vi "LearnBAGO.vi"(8 "error in (no error)":errorcluster, 11 "AER in":refnum<class "AER.lvclass">) -> (0 "error out":errorcluster, 3 "AER out":refnum<class "AER.lvclass">)   [LabVIEW 2016, in "AER.lvclass"]
uses:
  AER.lvclass
  AER.lvclass/AER.ctl
panel:
  out "size(s)":i32
  in  "gamma":dbl=-3e-05 format="%#_13g"
  out "WBAGO":dbl[](graph)
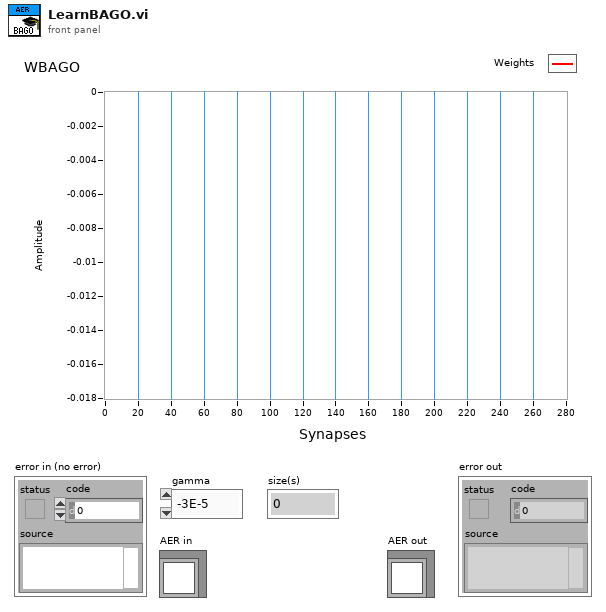
[diagram p1: front panel]
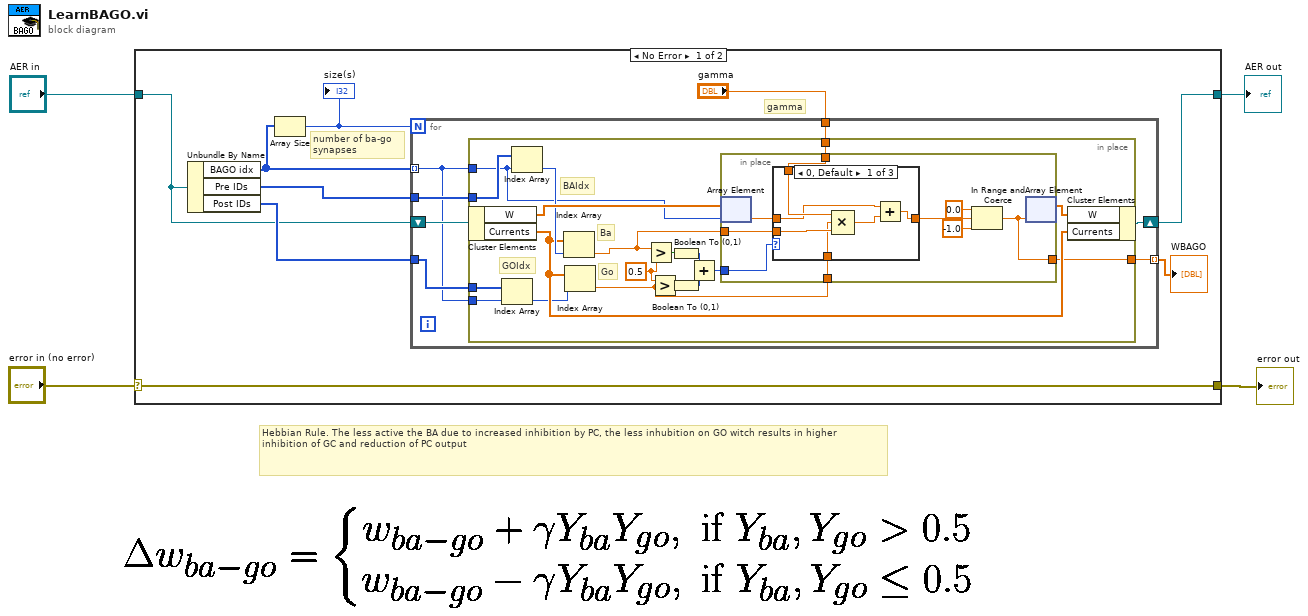
[diagram p0: block diagram]
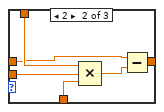
[diagram p2: hidden frame]
diagram:
  # "Hebbian Rule. The less active the BA due to increased inhibition by PC, the less inhubition on GO witch results in higher inhibition of GC and reduction of PC output"
  n1 = case shown="No Error" "error in (no error)" {
    selector: "error in (no error)" -> [w13 w62]
    tunnel: [w13 w62] -> w3
    tunnel: [w7 w63] -> w1
    tunnel: "AER in" -> [w6 w63]
    frame No Error {
      # "gamma"
      # "number of ba-go synapses"
      n2 = Unbundle By Name(w6) -> ("BAGO idx"=w11:i32[], "Pre IDs"=w10:i32[], "Post IDs"=w9:i32[])
      n3 = Array Size(array=w11) -> (size(s)=w12:i32)
      "size(s)" <- w12
      n4 = for {
        N: w12 -> [_]
        tunnel: w11 -> [w14] mode=indexing
        tunnel: w10 -> [w20]
        tunnel: w9 -> [w19]
        tunnel: "gamma" -> [w18]
        shift-right: [w17] -> w7
        shift-left: w6 -> [w16]
        tunnel: [w15] -> w5 mode=indexing
        n5 = in-place {
          in-place-border: w14 -> [w24]
          in-place-border: w20 -> [w39]
          in-place-border: w19 -> [w35]
          in-place-border: w18 -> [w29]
          in-place-border: [w27] -> w15
          in-place-border: w14 -> [w26]
          w23 = 0.5 ("x")
          # "GOIdx"
          # "Go"
          # "Ba"
          # "BAIdx"
          n6 = in-place-cluster #1(w16) -> ("W"=w38:dbl[], "Currents"=w36:dbl[])
          n7 = Index Array(array=w35, index=w26) -> (element=w25:i32)
          n8 = Index Array(array=w39, index=w24) -> (element=w37:i32)
          n9 = Index Array(array=w36, index=w37) -> (element=w22:dbl)
          n10 = Index Array(array=w36, index=w25) -> (element=w30:dbl)
          n11 = Greater?(x=w22, y=w23) -> (0:w21:bool)
          n12 = Greater?(x=w23, y=w30) -> (0:w34:bool)
          n13 = Boolean To (0,1)(Boolean=w21) -> (0, 1=w32:i16)
          n14 = Boolean To (0,1)(Boolean=w34) -> (0, 1=w31:i16)
          n15 = Add(x=w32, y=w31) -> (x+y=w33:i16)
          n16 = in-place {
            in-place-border: w33 -> [w48]
            in-place-border: w22 -> [w46]
            in-place-border: w30 -> [w45]
            in-place-border: w29 -> [w44]
            in-place-border: [w42] -> w27
            n17 = in-place-array #2(w38, w24) -> (w47:dbl)
            n18 = case shown="0, Default" w48 {
              tunnel: w47 -> [w50 w55 w61]
              tunnel: w46 -> [w54 w58 _]
              tunnel: w45 -> [w53 w57 _]
              tunnel: w44 -> [w52 w56 _]
              tunnel: [w49 w59 w61] -> w43
              frame 0, Default {
                n19 = Compound Arithmetic op=MULTIPLY(w52, w53, w54) -> (w51:dbl)
                n20 = Add(x=w50, y=w51) -> (x+y=w49:dbl)
              }
              frame 2 {
                n21 = Compound Arithmetic op=MULTIPLY(w56, w58, w57) -> (w60:dbl)
                n22 = Subtract(x=w55, y=w60) -> (x-y=w59:dbl)
              }
              frame 1 {
              }
            }
            n23 = In Range and Coerce(upper limit=0.0, x=w43, lower limit=-1.0) -> (coerced(x)=w42:dbl)  [unwired: 1 out]
            n24 = in-place-array #2(w42) -> (w28:dbl[])  [unwired: 1 out]
          }
          n25 = in-place-cluster #1("W"=w28, "Currents"=w36) -> (w17:refnum<class "AER.lvclass">)
        }
      }
      "WBAGO" <- w5
    }
    frame Error {
    }
  }
  "error out" <- w3
  "AER out" <- w1
